vi "GSI-HVSwitch2.read data.vi"(0 "i ref in":refnum<vi>, 3 "ms timeout (10000)":i32=10000, 5 "error in (no error)":errorcluster) -> (9 "ActTempAmp":dbl format="%.2f", 11 "ActTempPS1":dbl format="%.2f", 13 "ActTempPS2":dbl format="%.2f", 14 "i ref out":refnum<vi>, 15 "ActVoltage":dbl format="%.2f", 17 "timed out":bool, 19 "error out":errorcluster)   [LabVIEW 2014, in "GSI-HVSwitch2.lvlib"]
doc: "Reads the actual data from the instrument."
uses:
  GSI-HVSwitch2.lvlib
  CSCore/CSSystem/CoreDefs/CoreDefs.error_type.ctl
  CSinstr.lib/hvSwitch2/HVSwitch2Driver.lvlib
  CSCore/CSSystem/CoreLib/CoreLib.lvlib
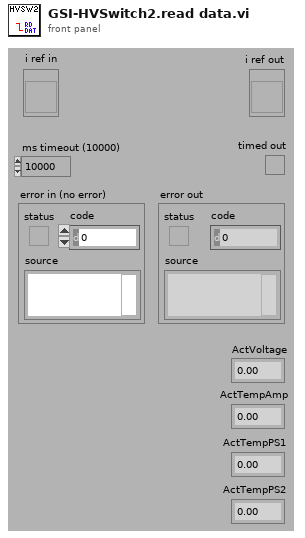
[diagram p1: front panel]
types:
  T1 = typedef "CoreDefs.error_type.ctl" = enum16{"no error", "can't load process", "can't unload process", "process does not exist", "can't install process", "can't remove process", "unknown function", "time out", "can't execute function", "duplicate queue name", "super not found", "caller queue invalid", "can't ping process", "unknown error", "VISA Error", "VISA timeout", "GPIB timeout", "GPIB error", "communication error", "data type mismatch", "can't read data from OPC server", "can't write data to OPC server", "OET error", "function not implemented", "process already exists", "invalid Shared Variable name", "error writing Shared Variable", "error reading Shared Variable", "invalid client name", "corrupt database", "unknown class", "call not authorized", "parameter out of range", "OET timeout: can't get data to modify", "invalid queue name", "requested operation incompatible with current state", "event undefined", "event disabled", "state undefined", "caller is not a friend", "EventBuilder: bad eventID", "EventBuilder: no DAQ devices", "a thread must not stop itself", "UNUSED ELEMENT4", "DiscArchiver: eventData incomplete", "DiscArchiver: eventData does not belong to run", "DiscArchiver: can't open file", "DiscArchiver: can't write to file", "DiscArchiver: available disc space low", "can't acquire semaphore", "error reading data from database", "notifier object is not existing", "can't register process", "can't unregister process", "illegal event type", "object disabled", "object already exists", "can't change state", "Instrument not found", "no connection to remote node", "invalid reference", "N/A", "UNUSED ELEMENT 1", "element not found", "illegal TCP/IP connection detected", "object does not exist", "invalid access ID", "unknown CS system", "invalid privilige", "unsupported data type", "unsupported server type", "IO server already exists", "Shared Variable already exists"}
  T2 = typedef "SDEXDriver.lvlib/SDEX.VISA Control.ctl" = cluster{"VISA resource name":refnum<visa-resource-name>, "HEX address":u16, "VISA Timeout Value (1000 ms)":u32, "Lock Timeout (1000 ms)":u32, "semaphore":T3, "Baud rate":u32, "revision":T4, "deviceInfo":string}
  T3 = typedef "Semaphore RefNum" = refnum<k1>
  T4 = typedef "SDEXDriver.lvlib/SDEX.revisionType.ctl" = enum16{"unknown", "hvamp3", "hvswi1", "htrp0", "WDG0"}
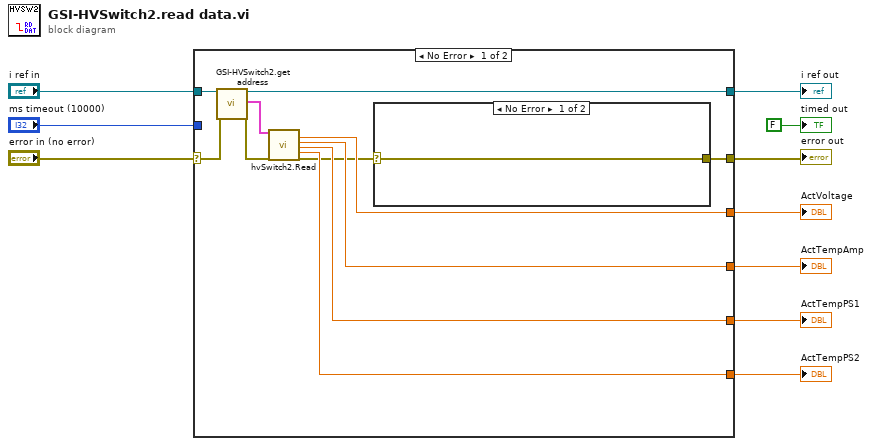
[diagram p0: block diagram]
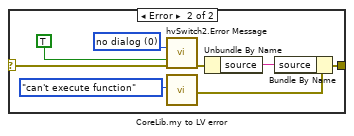
[diagram p2: hidden frame]
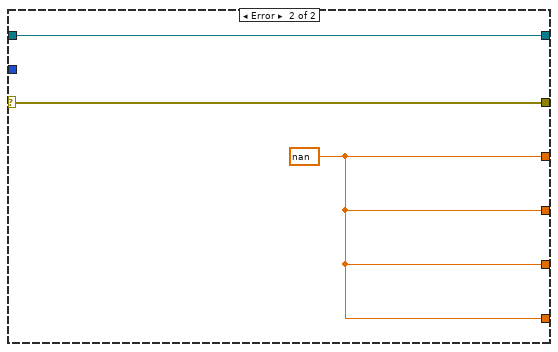
[diagram p3: hidden frame]
diagram:
  n1 = case shown="No Error" "error in (no error)" {
    selector: "error in (no error)" -> [w14 w33]
    tunnel: [w21 w33] -> w10
    tunnel: "i ref in" -> [w15 w32]
    tunnel: [w20 w31] -> w8
    tunnel: [w19 w31] -> w7
    tunnel: [w18 w31] -> w6
    tunnel: [w17 w31] -> w5
    tunnel: [w11 w32] -> w2
    tunnel: "ms timeout (10000)" -> [_ _]
    frame No Error {
      n2 = call "GSI-HVSwitch2.get address.vi"("i ref in"=w15, "error in (no error)"=w14) -> ("i ref out"=w11:refnum<vi>, "SDEX address"=w12:T2, "error out"=w13:errorcluster)  [unwired: 15 in]
      n3 = call "hvSwitch2.Read.vi"("SDEX VISA Cluster"=w12, "error in (no error)"=w13) -> ("ActVoltage"=w20:dbl, "ActTempAmp"=w19:dbl, "ActTempPS1"=w18:dbl, "ActTempPS2"=w17:dbl, "error out"=w16:errorcluster)  [unwired: 12 in, 1 out]
      n4 = case shown="No Error" w16 {
        selector: w16 -> [w22 w28]
        tunnel: [w22 w26] -> w21
        frame No Error {
        }
        frame Error {
          w30 = u16 0 items=["no dialog", "OK message", "continue or stop message"] ("type of dialog (no dialog: 0)")
          n5 = call "hvSwitch2.Error Message.vi"("Type of Dialog (0: No Dialog)"=w30, "append msg 2 src"=TRUE ("add message to source"), "error in (no error)"=w28) -> ("error out"=w24:errorcluster)  [unwired: 8 in, 4 out]
          n6 = call "CoreLib.my to LV error.vi"("ErrorTypes"=CoreDefs.error_type."can't execute function") -> ("myErrorCluster"=w25:errorcluster)  [unwired: 17 in, 1 out]
          n7 = Unbundle By Name(w24) -> ("source"=w23:string)
          n8 = Bundle By Name(cluster=w25, "source"=w23) -> (w26:errorcluster)
        }
      }
    }
    frame Error {
      w31 = nan ("ActVoltage")
    }
  }
  "error out" <- w10
  "i ref out" <- w2
  "ActVoltage" <- w8
  "ActTempAmp" <- w7
  "ActTempPS1" <- w6
  "ActTempPS2" <- w5
  "timed out" <- FALSE ("timed out")
